vi "close connection.vi"(8 "error in (no error)":errorcluster, 11 "DeviceInterface in":refnum<class "DeviceInterface.lvclass">) -> (0 "error out":errorcluster, 3 "DeviceInterface out":refnum<class "DeviceInterface.lvclass">)   [LabVIEW 2013, in "DeviceInterface.lvclass"]
doc: "Visa-Verbindung mit dem Gerät schliessen."
uses:
  DeviceInterface.lvclass
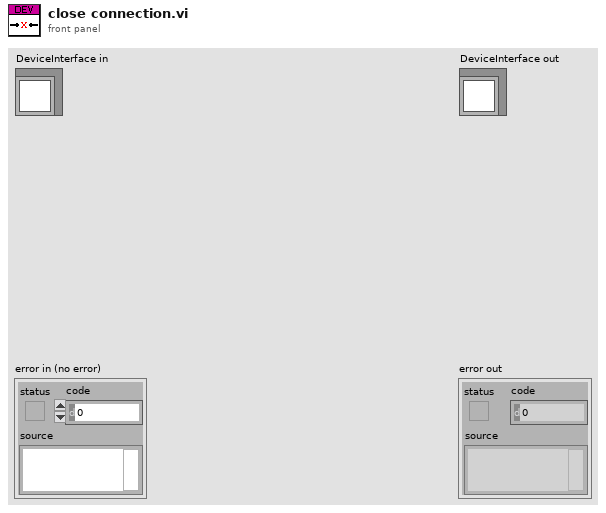
[diagram p1: front panel]
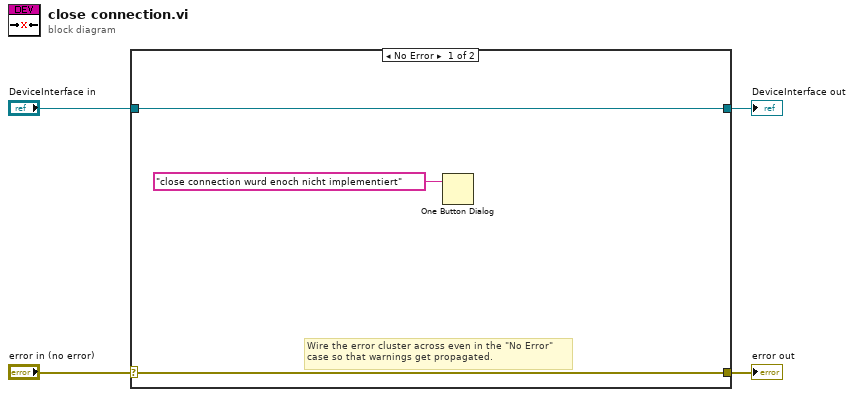
[diagram p0: block diagram]
diagram:
  n1 = case shown="No Error" "error in (no error)" {
    selector: "error in (no error)" -> [w6 w9]
    tunnel: [w6 w9] -> w3
    tunnel: [w7 w8] -> w1
    tunnel: "DeviceInterface in" -> [w7 w8]
    frame No Error {
      # "Wire the error cluster across even in the \"No Error\"\ncase so that warnings get propagated."
      n2 = One Button Dialog(message="close connection wurd enoch nicht implementiert") -> ()  [unwired: 1 in, 1 out]
    }
    frame Error {
    }
  }
  "error out" <- w3
  "DeviceInterface out" <- w1
